vi "Convert dB to percentage.vi"() -> ()   [LabVIEW 2016]
panel:
  in  "dB":dbl=-9.0 format="%#_13g"
  out "%":dbl
  out "exp(x)":dbl
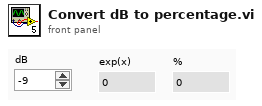
[diagram p1: front panel]
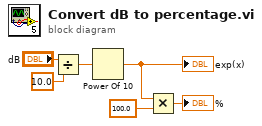
[diagram p0: block diagram]
diagram:
  n1 = Divide(x="dB", y=10.0) -> (x/y=w4:dbl)
  n2 = Power Of 10(x=w4) -> (10^x=w3:dbl)
  "exp(x)" <- w3
  n3 = Multiply(x=w3, y=100.0) -> (x*y=→"%":dbl)
